vi "Random (SubVI).vi"(11 "Input":i32[][](array[numeric])) -> (3 "Output":i32[][](array[numeric]))   [LabVIEW 2020]
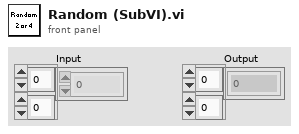
[diagram p1: front panel]
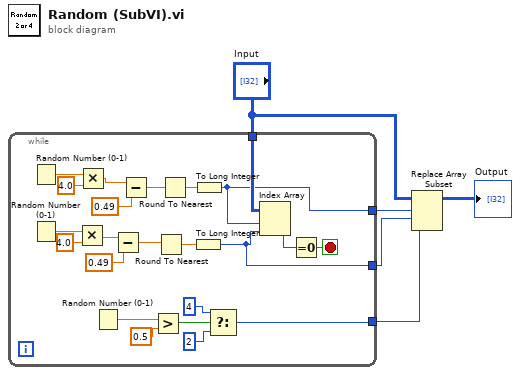
[diagram p0: block diagram]
diagram:
  n1 = while {
    tunnel: "Input" -> [w17]
    tunnel: [w15] -> w2
    tunnel: [w14] -> w3
    tunnel: [w13] -> w4
    stop <- w18 stop-if-true
    n2 = Random Number (0-1)() -> (number: 0 to 1=w19:dbl)
    n3 = Random Number (0-1)() -> (number: 0 to 1=w12:dbl)
    n4 = Multiply(x=w12, y=4.0) -> (x*y=w10:dbl)
    n5 = Multiply(x=w19, y=4.0) -> (x*y=w11:dbl)
    n6 = Random Number (0-1)() -> (number: 0 to 1=w24:dbl)
    n7 = Subtract(x=w10, y=0.49) -> (x-y=w9:dbl)
    n8 = Subtract(x=w11, y=0.49) -> (x-y=w8:dbl)
    n9 = Greater?(x=w24, y=0.5) -> (0:w27:bool)
    n10 = Round To Nearest(number=w9) -> (nearest integer value=w22:dbl)
    n11 = Round To Nearest(number=w8) -> (nearest integer value=w21:dbl)
    n12 = To Long Integer(number=w22) -> (32bit integer=w13:i32)
    n13 = To Long Integer(number=w21) -> (32bit integer=w14:i32)
    n14 = Select(t=4 ("index (row)"), s=w27, f=2 ("index (row)")) -> (s? t:f=w15:i32)
    n15 = Index Array(array=w17, index (row)=w14, index (col)=w13) -> (element=w16:i32)
    n16 = Equal To 0?(x=w16) -> (x = 0?=w18:bool)
  }
  n17 = Replace Array Subset(array="Input", new element=w2, index (row)=w3, index (col)=w4) -> (→"Output":i32[][])
